vi "Find Center.vi"(7 "Tray Number":dbl format="%#_13g", 9 "XYZTheta":dbl[](array[numeric]), 11 "Gantry In":refnum<k24>) -> (1 "XYZTheta Centers":dbl[][](array[numeric]), 3 "Gantry Out":refnum<k24>)   [LabVIEW 2021, in "Assembly Tray.lvclass"]
uses:
  Assembly Tray.lvclass
  Find Tray.ctl
  Controller/Camera/Machine Vision.ctl
  C:/Program Files (x86)/Aerotech/A3200/LabVIEW/2010/Bin/Aerotech.A3200.dll
  Program Files (x86)/Aerotech/A3200/LabVIEW/2010/Bin/Aerotech.A3200.dll
  Controller/Camera/Image processing.ctl
  Controller/Camera/Camera settings.ctl
  Controller/Camera/Material.ctl
  Program Files (x86)/National Instruments/LabVIEW 2021/examples/Connectivity/Python/support/PythonVersionsEnum.ctl
  Controller/Camera/Camera.lvclass
  Controller/Motion/A3200/A3200.lvclass
  Controller/Motion/Motion.lvclass
panel:
  out "Move by":dbl[](array[numeric])
  in  "Autofiducial (Beta)":bool
  in  "Focus step size":dbl format="%#_13g"
  in  "number of focus steps":i32
  out "Average Strength":dbl
  in  "Focus":bool
  in  "Material":T1
  in  "Camera settings":T2={"Gamma"=1.6, "Gain"=0, "Sharpness"=0, "Contrast"=0.0, "Exposure"=0.0078125} {"Exposure" min=0.000244140625 max=0.5 scale=0.0002..0.5; "Contrast" min=0.0 max=1.0 scale=0.001..1.0; "Sharpness" min=0 max=2 step=1 scale=0.0..2.0; "Gain" min=0 max=100 step=1 scale=0.1..100.0; "Gamma" min=0.01 max=10.0 scale=0.01..10.0}
  in  "Image processing":T3={"Brightness"=128.0, "Contrast"=45.0, "Gamma"=1.0471123} {"Brightness" scale=0.0..400.0; "Contrast" scale=0.0..90.0; "Gamma" scale=0.005..5.0}
  in  "Override presets":bool
  out "Both fiducials recorded":bool
  in  "Machine Vision":T4
  out "Right Fiducial":dbl[](array[numeric]) format="%.6g"
  out "Left Fiducial":dbl[](array[numeric]) format="%.6g"
  out "Gantry":dbl[](array[numeric]) format="%.6g"
  out "Sum":dbl[](array[numeric]) format="%.6g"
  out "Camera":dbl[](array[numeric]) format="%.6g"
  in  "Carrier Tray":T5
  out "Image":T6(plugin-control)
  out "Center":dbl[](array[numeric]) format="%.6g"
  in  "Position Number":i16
  in  "Go to Center":bool
  in  "Calculate":bool
  in  "Record Bottom":bool
  in  "Record Top":bool
  in  "Go to Bottom Fiducial":bool
  in  "Go to Top Fiducial":bool
  in  "Joystick":bool
  in  "Stop":bool
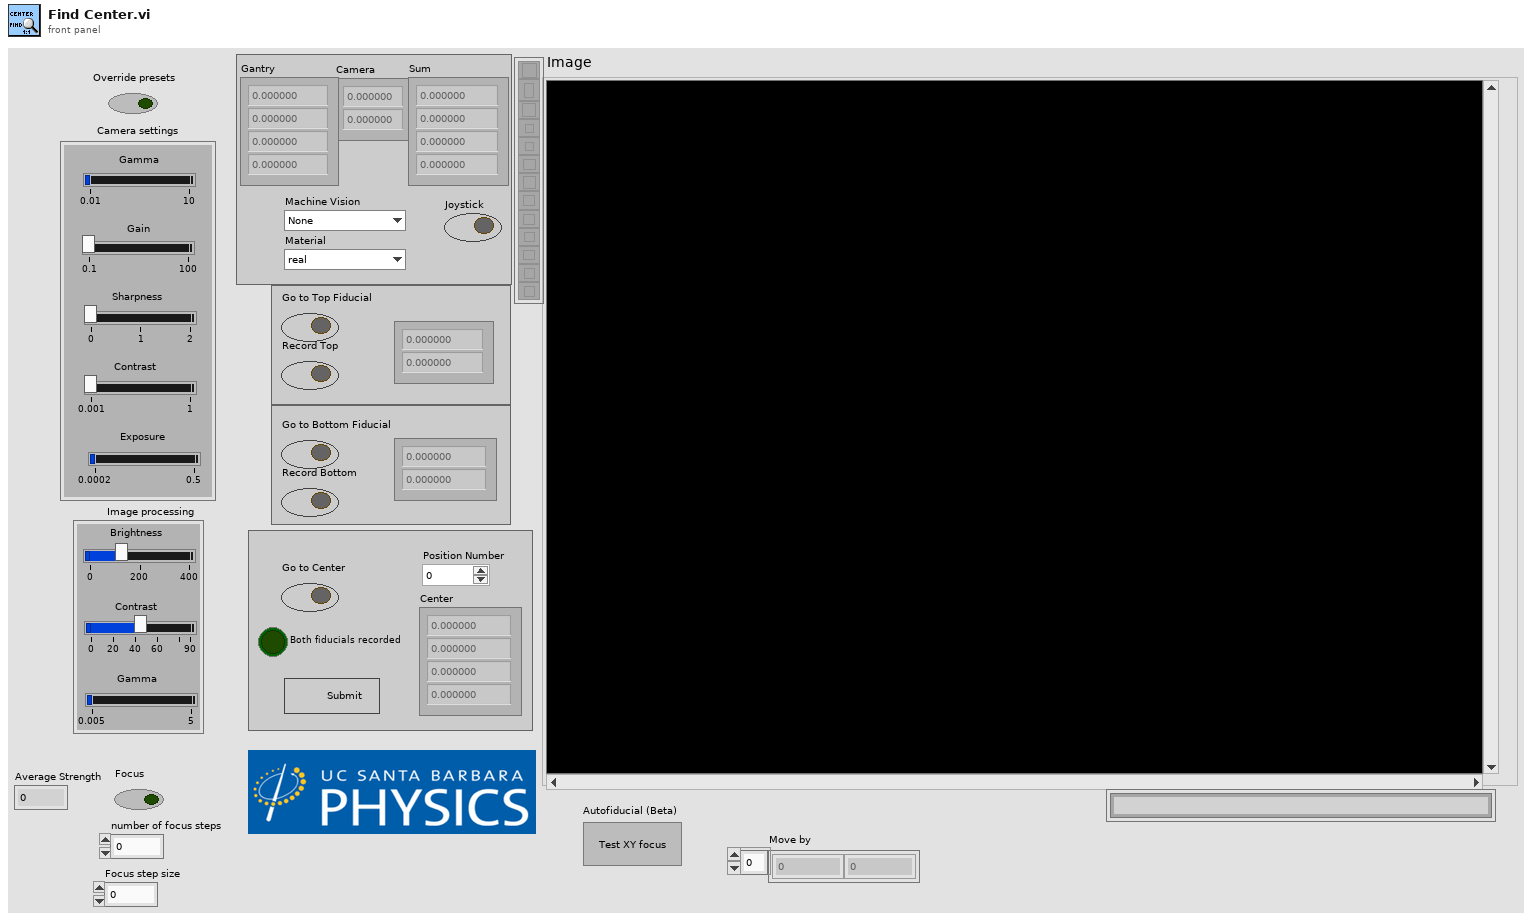
[diagram p1: front panel]
types:
  T1 = typedef "Camera.lvclass/Material.ctl" = enum16{"real", "dummy", "PETG"}
  T2 = typedef "Camera.lvclass/Camera settings.ctl" = cluster{"Gamma":dbl, "Gain":i64, "Sharpness":i64, "Contrast":dbl, "Exposure":dbl}
  T3 = typedef "Camera.lvclass/Image processing.ctl" = cluster{"Brightness":sgl, "Contrast":sgl, "Gamma":sgl}
  T4 = typedef "Camera.lvclass/Machine Vision.ctl" = enum16{"None", "Tray Fiducials", "HPK Silicon", "100um dot", "Hexaboard", "Corner (TL, BR)", "Corner (BL, TR)", "BP gold pad 1", "BP gold pad 2", "BP gold pad 3", "dummy sensor CH2", "dummy sensor CH7", "dummy sensor CH191", "dummy sensor CH197", "sensor box", "sensor circle", "PCB PETG CH2", "PCB PETG CH7", "PCB PETG CH191", "PCB PETG CH197"}
  T5 = typedef "Assembly Tray.lvclass/Find Tray.ctl" = cluster{"Gantry Fiducials":dbl[], "Relative Coordinates":dbl[][], "Camera Fiducials":dbl[][], "XYZTheta Centers":dbl[][], "Workspace Center":dbl[], "Syringe Relative Coordinates":dbl[], "Gantry Region":dbl, "Fiducials":path, "New Fiducials":dbl[][], "Past Fiducials":dbl[][], "XYZTheta":dbl[], "Position":dbl}
  T6 = typedef "IMAQ Image.ctl" = refnum<image>
  T7 = typedef "PythonVersionsEnum.ctl" = enum16{"3.6", "3.7", "3.8", "3.9"}
  T8 = typedef "File Paths.ctl" = cluster{"Glue Pattern Folder":path, "Carrier Tray Folder":path, "Pick Up Tool Fixture Folder":path, "Components Folder":path, "Bellows Tool Offset.txt":path, "Pick Up Tool Offset.txt":path, "Dispense Tip Offset.txt":path, "Log Files":path, "Gantry Assembly Map.txt":path, "Syringe and offset map.txt":path}
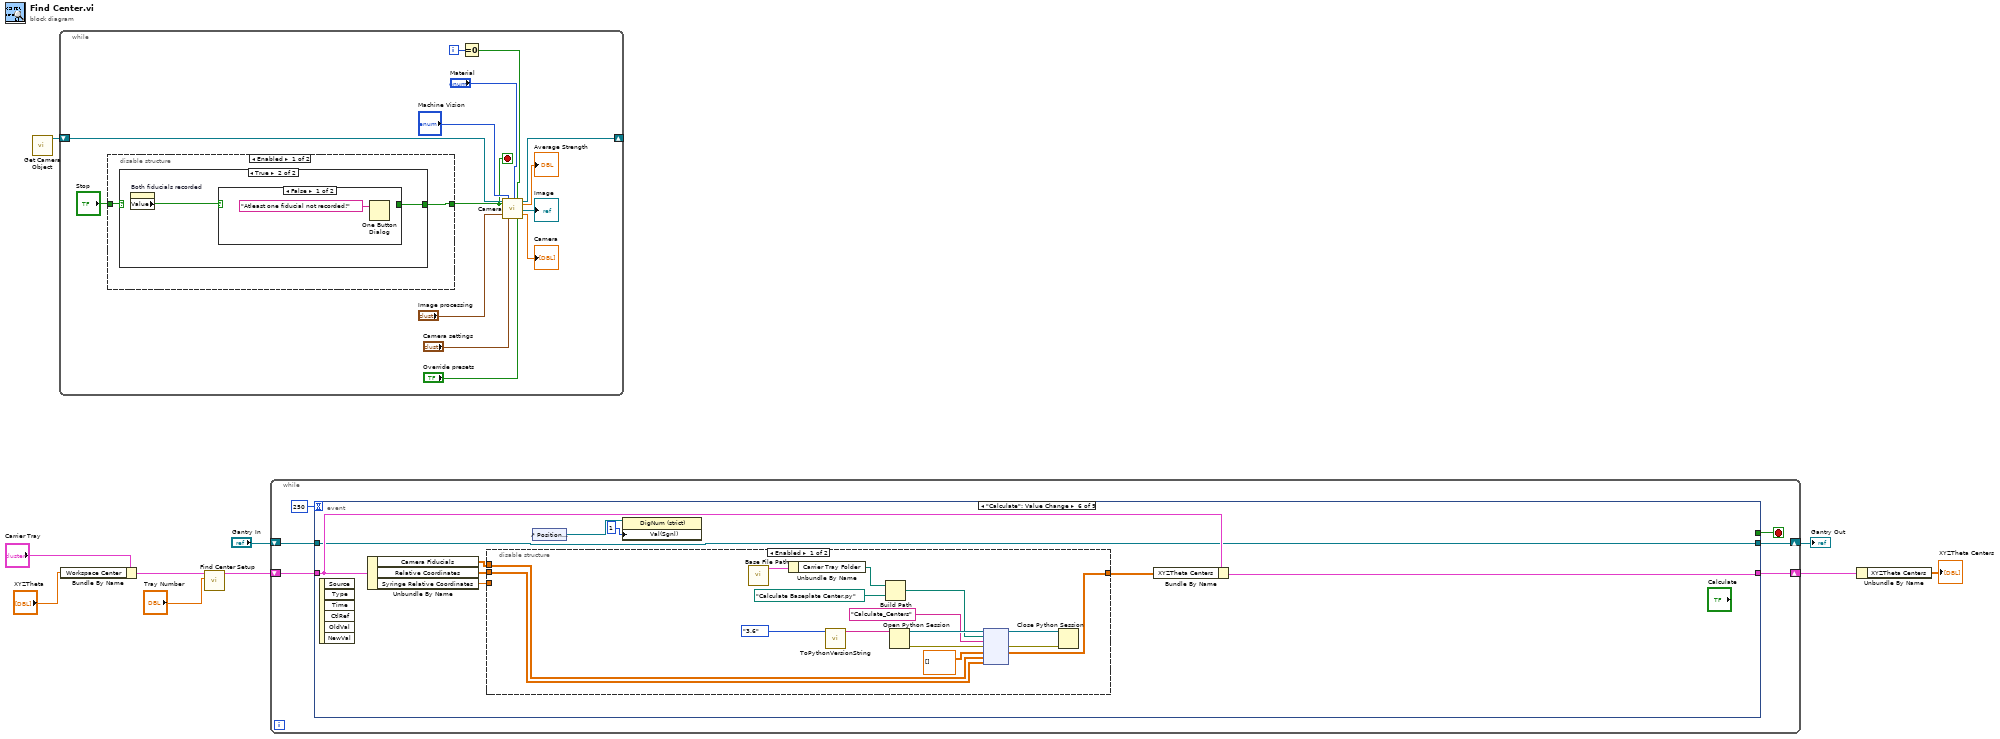
[diagram p0: block diagram]
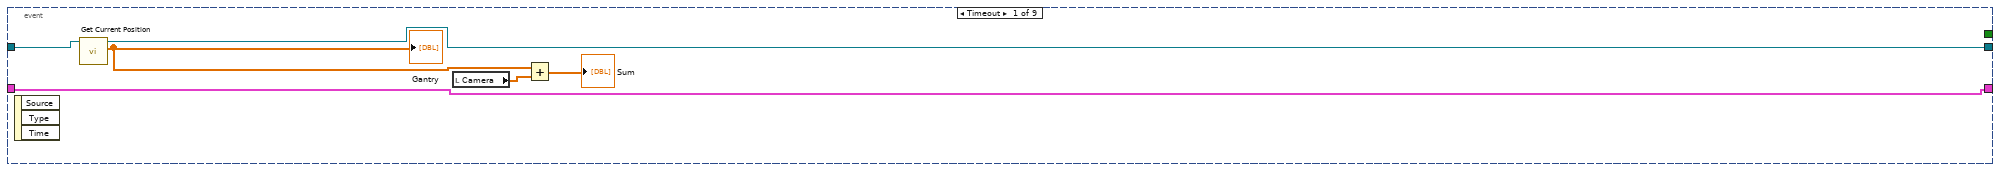
[diagram p2: hidden frame]
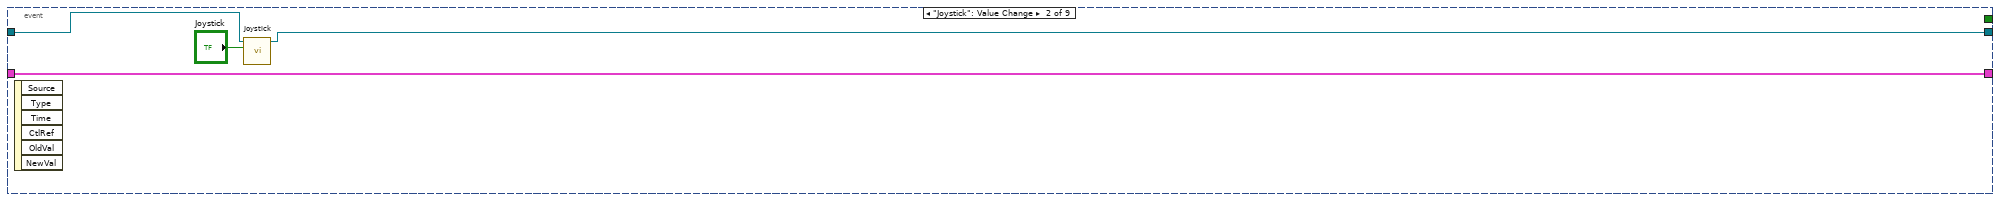
[diagram p3: hidden frame]
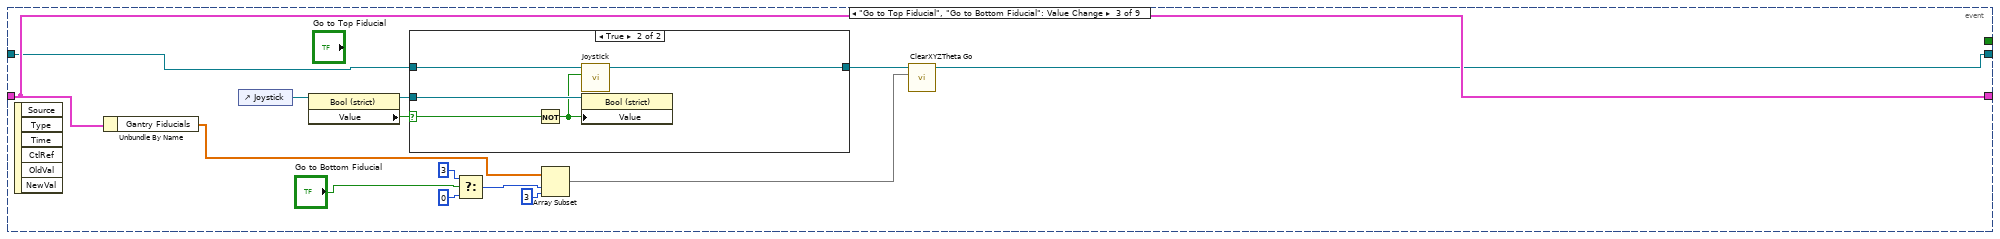
[diagram p4: hidden frame]
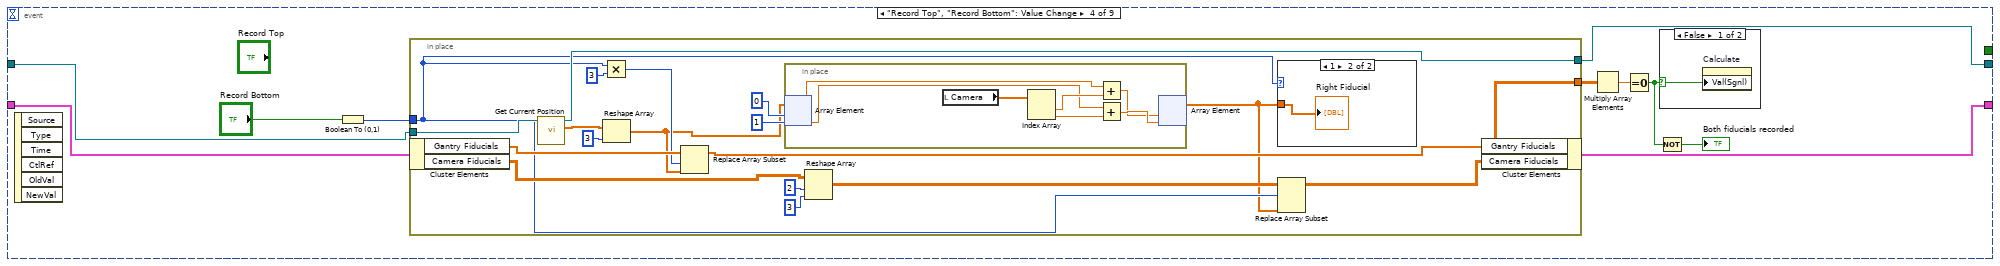
[diagram p6: hidden frame]
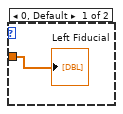
[diagram p8: hidden frame]
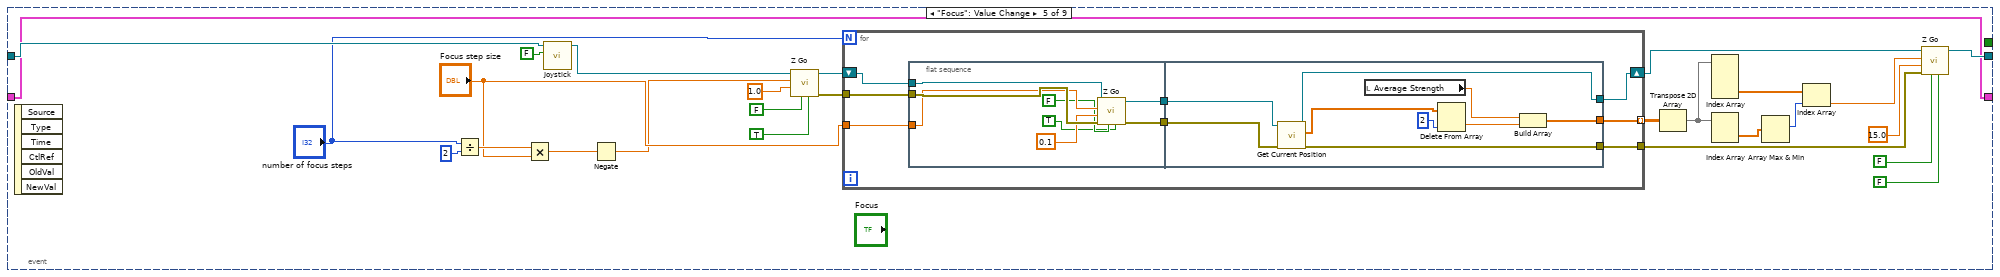
[diagram p9: hidden frame]
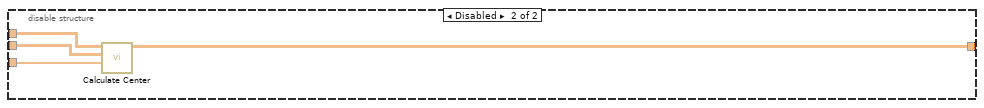
[diagram p10: hidden frame]
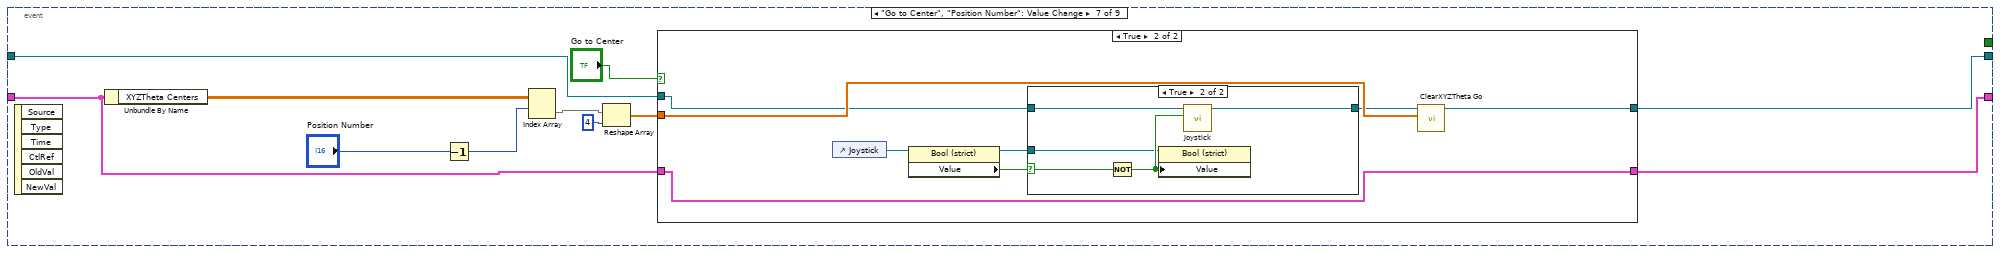
[diagram p11: hidden frame]
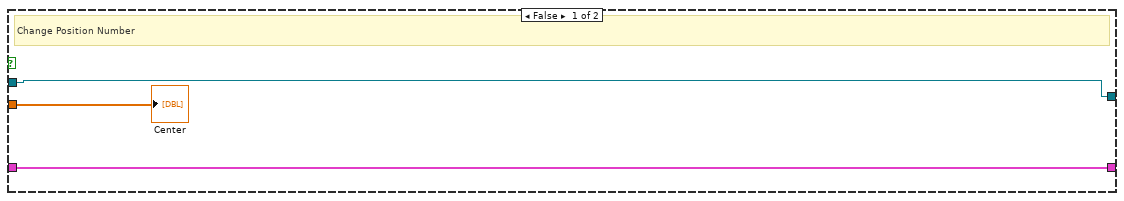
[diagram p12: hidden frame]
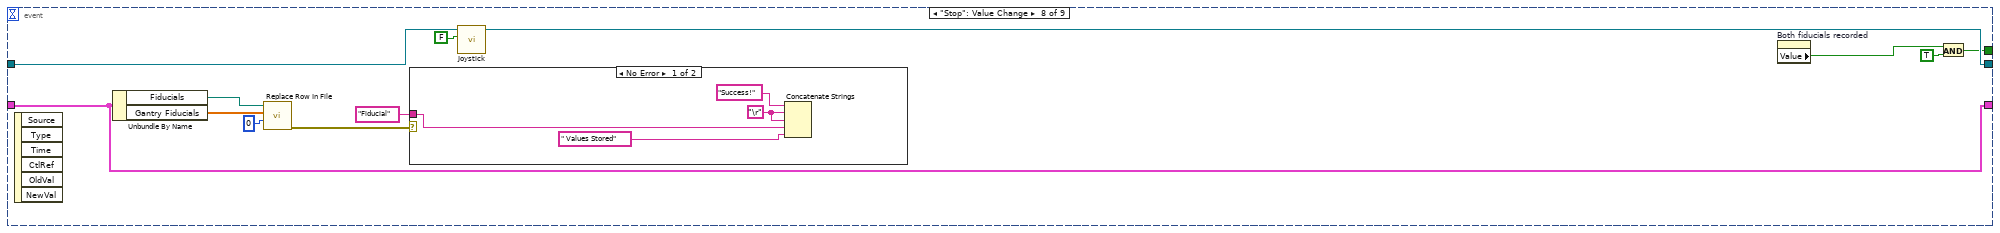
[diagram p14: hidden frame]
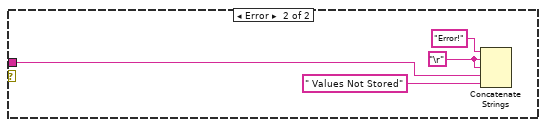
[diagram p15: hidden frame]
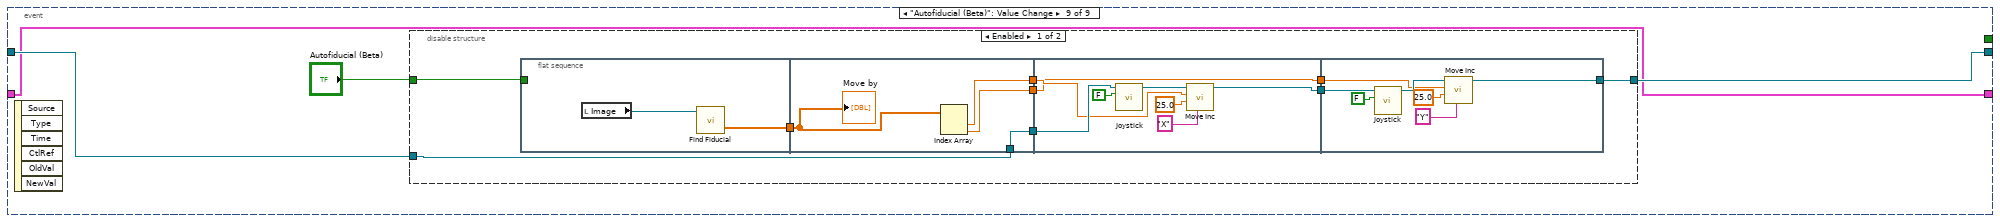
[diagram p16: hidden frame]
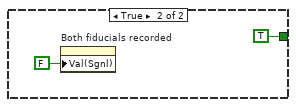
[diagram p19: hidden frame]
diagram:
  n1 = call "Get Camera Object.vi"() -> ("Camera out"=w4:refnum<class "Camera.lvclass">)  [unwired: 10 in, 1 out]
  n2 = while {
    shift-right: [w20] -> _
    shift-left: w4 -> [w24]
    i -> [w14]
    stop <- w19 stop-if-true
    n3 = disable-structure shown="Enabled" {
      disable-tunnel: [w25 w32] -> w19
      disable-tunnel: "Stop" -> [w26 w32]
      frame Enabled {
        n4 = case shown="True" w26 {
          tunnel: [_ w27] -> w25
          frame False {
          }
          frame True {
            n5 = property on="Both fiducials recorded" class="Bool (strict)"() -> ("Value"=w28:bool)  [unwired: 2 in, 2 out]
            n6 = case shown="False" w28 {
              tunnel: [_ TRUE] -> w27
              frame False {
                n7 = One Button Dialog(message="Atleast one fiducial not recorded!") -> ()  [unwired: 1 in, 1 out]
              }
              frame True {
                n8 = property on="Both fiducials recorded" class="Bool (strict)"("Val(Sgnl)"=FALSE) -> ()  [unwired: 2 in, 2 out]
              }
            }
          }
        }
      }
      frame Disabled {
      }
    }
    n9 = Equal To 0?(x=w14) -> (x = 0?=w13:bool)
    n10 = call "Camera.vi"("Camera in"=w24, "Stop"=w19, "BCG Image Processing"="Image processing", "Machine Vision"="Machine Vision", "Camera settings"="Camera settings", "Material"="Material", "Loop 0"=w13, "Override presets"="Override presets") -> ("Camera out"=w20:refnum<class "Camera.lvclass">, "Average Strength"=→"Average Strength":dbl, "Image"=→"Image":T6, "Camera"=→"Camera":dbl[])  [unwired: 5 in, 3 out]
  }
  n11 = Bundle By Name(cluster="Carrier Tray", "Workspace Center"="XYZTheta") -> (w7:T5)
  n12 = call "Find Center Setup.vi"("Carrier Tray"=w7, "Tray Number"="Tray Number") -> ("Assembly Tray Out"=w10:T5)  [unwired: 8 in]
  n13 = while {
    shift-right: [w37] -> w9
    shift-left: w10 -> [w38]
    shift-right: [w33] -> w2
    shift-left: "Gantry In" -> [w34]
    stop <- w36 stop-if-true
    n14 = event shown="[5] \"Calculate\": Value Change" {
      selector: _ -> [_ _ _ _ _ _ _ _ _]
      dyn-events: _ -> [_ _ _ _ _ _ _ _ _]
      timeout: 250 -> [_ _ _ _ _ _ _ _ _]
      tunnel: [w42 w48 w62 w78 w118 w164 w194 w222 w235] -> w37
      tunnel: w38 -> [w42 w48 w62 w73 w118 w165 w195 w222 w235]
      tunnel: [_ _ _ _ _ _ _ w217 _] -> w36
      tunnel: w34 -> [w41 w47 w54 w72 w120 w163 w192 w223 w237]
      tunnel: [w39 w45 w51 w71 w119 w163 w188 w218 w238] -> w33
      event Timeout {
        n15 = event-data() -> ()  [unwired: 1 in, 3 out]
        n16 = call "Get Current Position.vi"("Gantry In"=w41) -> ("XYZTheta Out"=w40:dbl[], "Gantry Out"=w39:refnum<k24>)  [unwired: 8 in, 1 out]
        "Gantry" <- w40
        n17 = local read "Camera"() -> (w44:dbl[])
        n18 = Add(x=w40, y=w44) -> (x+y=→"Sum":dbl[])
      }
      event "Joystick": Value Change {
        n19 = event-data() -> ()  [unwired: 1 in, 6 out]
        n20 = call "Joystick.vi"("Joystick"="Joystick", "Gantry In"=w47) -> ("Gantry Out"=w45:refnum<k24>)  [unwired: 8 in, 1 out]
      }
      event "Go to Top Fiducial", "Go to Bottom Fiducial": Value Change {
        n21 = event-data() -> ()  [unwired: 1 in, 6 out]
        n22 = Unbundle By Name(w62) -> ("Gantry Fiducials"=w50:dbl[])
        n23 = control-ref of="Joystick"() -> (w61:refnum<vi>)
        n24 = property class="Bool (strict)"(reference=w61) -> (reference out=w52:refnum<vi>, "Value"=w55:bool)  [unwired: 1 in, 1 out]
        n25 = case shown="True" w55 {
          selector: w55 -> [_ w68]
          tunnel: w54 -> [w63 w66]
          tunnel: [w63 w65] -> w53
          tunnel: w52 -> [_ w67]
          frame False {
          }
          frame True {
            n26 = Not(x=w68) -> (.not. x?=w64:bool)
            n27 = call "Joystick.vi"("Joystick"=w64, "Gantry In"=w66) -> ("Gantry Out"=w65:refnum<k24>)  [unwired: 8 in, 1 out]
            n28 = property class="Bool (strict)"(reference=w67, "Value"=w64) -> ()  [unwired: 1 in, 2 out]
          }
        }
        n29 = Select(t=3, s="Go to Bottom Fiducial", f=0) -> (s? t:f=w59:i32)
        n30 = Array Subset(array=w50, index=w59, length=3) -> (w49:dbl[])
        n31 = call "ClearXYZTheta Go.vi"("XYZTheta In"=w49, "Gantry In"=w53) -> ("Gantry Out"=w51:refnum<k24>)  [unwired: 7 in, 2 out]
      }
      event "Record Top", "Record Bottom": Value Change {
        n32 = event-data() -> ()  [unwired: 1 in, 6 out]
        n33 = Boolean To (0,1)(Boolean="Record Bottom") -> (0, 1=w75:i16)
        n34 = in-place {
          in-place-border: [w91] -> w76
          in-place-border: w75 -> [w84]
          in-place-border: w72 -> [w86]
          in-place-border: [w85] -> w71
          n35 = in-place-cluster #1(w73) -> ("Gantry Fiducials"=w88:dbl[], "Camera Fiducials"=w95:dbl[][])
          n36 = call "Get Current Position.vi"("Gantry In"=w86) -> ("XYZTheta Out"=w89:dbl[], "Gantry Out"=w85:refnum<k24>)  [unwired: 8 in, 1 out]
          n37 = Multiply(x=w84, y=i16 3) -> (x*y=w82:i16)
          n38 = Reshape Array(w89, 3 ("dimension size")) -> (w81:dbl[])
          n39 = Replace Array Subset(array=w88, new element=w81, index=w82) -> (w87:dbl[])
          n40 = in-place {
            n41 = in-place-array #2(w81, 0, 1) -> (w103:dbl, w101:dbl)
            n42 = local read "Camera"() -> (w104:dbl[])
            n43 = Index Array(array=w104) -> (element #1=w102:dbl, element #2=w100:dbl)  [unwired: 2 in]
            n44 = Add(x=w103, y=w102) -> (x+y=w98:dbl)
            n45 = Add(x=w101, y=w100) -> (x+y=w99:dbl)
            n46 = in-place-array #2(w98, w99) -> (w80:dbl[])  [unwired: 2 out]
          }
          n47 = Reshape Array(w95, 2 ("length"), 3 ("dimension size")) -> (w94:dbl[][])
          n48 = case shown="1" w84 {
            tunnel: w80 -> [w105 w106]
            frame 0, Default {
              "Left Fiducial" <- w105
            }
            frame 1 {
              "Right Fiducial" <- w106
            }
          }
          n49 = Replace Array Subset(array=w94, new element=w80, index (row)=w84) -> (w91:dbl[][])  [unwired: 1 in]
          n50 = in-place-cluster #1("Gantry Fiducials"=w87, "Camera Fiducials"=w91) -> (w78:T5)
        }
        n51 = Multiply Array Elements(1:w76) -> (0:w77:dbl)
        n52 = Equal To 0?(x=w77) -> (x = 0?=w70:bool)
        n53 = Not(x=w70) -> (.not. x?=→"Both fiducials recorded":bool)
        n54 = case shown="False" w70 {
          selector: w70 -> [w79 _]
          frame False {
            n55 = property on="Calculate" class="Bool (strict)"("Val(Sgnl)"=w79) -> ()  [unwired: 2 in, 2 out]
          }
          frame True {
          }
        }
      }
      event "Focus": Value Change {
        n56 = event-data() -> ()  [unwired: 1 in, 6 out]
        n57 = Divide(x="number of focus steps", y=2) -> (x/y=w122:dbl)
        n58 = Multiply(x=w122, y="Focus step size") -> (x*y=w121:dbl)
        n59 = call "Joystick.vi"("Joystick"=FALSE, "Gantry In"=w120) -> ("Gantry Out"=w114:refnum<k24>)  [unwired: 8 in, 1 out]
        n60 = Negate(x=w121) -> (-x=w112:dbl)
        n61 = call "Z Go.vi"("Increment"=TRUE, "Return Immediately"=FALSE ("Increment"), "Speed In"=1.0 ("Speed"), "Position In"=w112, "Gantry In"=w114) -> ("error out"=w109:errorcluster, "Gantry Out"=w113:refnum<k24>)  [unwired: 3 in, 2 out]
        n62 = for {
          N: "number of focus steps" -> [_]
          tunnel: [w138] -> w132 mode=indexing
          tunnel: w109 -> [w137]
          tunnel: [w135] -> w125
          shift-right: [w139] -> w126
          shift-left: w113 -> [w141]
          tunnel: "Focus step size" -> [w134]
          n63 = flat-sequence {
            tunnel: w141 -> [w149]
            tunnel: [w148] -> w140
            tunnel: w137 -> [w146]
            tunnel: [w147] -> w136
            tunnel: w134 -> [w144]
            tunnel: w140 -> [w158]
            tunnel: [w157] -> w139
            tunnel: [w156] -> w138
            tunnel: w136 -> [w152]
            tunnel: [w151] -> w135
            frame #0 {
              n64 = call "Z Go.vi"("Increment"=TRUE, "Return Immediately"=FALSE ("Increment"), "error in (no error)"=w146, "Speed In"=0.1 ("Speed"), "Position In"=w144, "Gantry In"=w149) -> ("error out"=w147:errorcluster, "Gantry Out"=w148:refnum<k24>)  [unwired: 2 in, 2 out]
            }
            frame #1 {
              n65 = call "Get Current Position.vi"("error in (no error)"=w152, "Gantry In"=w158) -> ("error out"=w151:errorcluster, "XYZTheta Out"=w155:dbl[], "Gantry Out"=w157:refnum<k24>)  [unwired: 7 in]
              n66 = local read "Average Strength"() -> (w150:dbl)
              n67 = Delete From Array(array=w155, index=2) -> (deleted portion=w153:dbl)  [unwired: 1 in, 1 out]
              n68 = Build Array(w150, w153) -> (w156:dbl[])
            }
          }
        }
        n69 = Transpose 2D Array(2D array=w132) -> (transposed array=w131:dbl[][])
        n70 = Index Array(array=w131) -> (element #2=w130:dbl[])  [unwired: 4 in, 1 out]
        n71 = Index Array(array=w131) -> (element=w133:dbl[])  [unwired: 2 in]
        n72 = Array Max & Min(array=w133) -> (max index (indices)=w129:i32)  [unwired: 3 out]
        n73 = Index Array(array=w130, index=w129) -> (element=w128:dbl)
        n74 = call "Z Go.vi"("Increment"=FALSE, "Return Immediately"=FALSE ("Increment"), "error in (no error)"=w125, "Speed In"=15.0 ("Speed"), "Position In"=w128, "Gantry In"=w126) -> ("Gantry Out"=w119:refnum<k24>)  [unwired: 2 in, 3 out]
      }
      event "Calculate": Value Change {
        n75 = event-data() -> ()  [unwired: 1 in, 6 out]
        n76 = Unbundle By Name(w165) -> ("Camera Fiducials"=w160:dbl[][], "Relative Coordinates"=w161:dbl[][], "Syringe Relative Coordinates"=w162:dbl[])
        n77 = disable-structure shown="Enabled" {
          disable-tunnel: w160 -> [w171 w185]
          disable-tunnel: w161 -> [w168 w184]
          disable-tunnel: w162 -> [_ w183]
          disable-tunnel: [w172 w186] -> w159
          frame Enabled {
            n78 = call "Base File Path.vi"() -> ("Paths Out"=w170:T8)  [unwired: 11 in]
            n79 = Unbundle By Name(w170) -> ("Carrier Tray Folder"=w169:path)
            n80 = call "ToPythonVersionString.vi"("python version"=PythonVersionsEnum."3.6") -> ("python version string"=w181:string)  [unwired: 10 in]
            n81 = Build Path(base path=w169, name or relative path=path "Calculate Baseplate Center.py") -> (appended path=w174:path)
            n82 = Open Python Session(python version=w181) -> (session out=w180:refnum<k35>, error out=w178:errorcluster)  [unwired: 2 in]
            n83 = node(w180, w174, "Calculate_Centers" ("function name"), w178, dbl[][] [], w171, w168) -> (w179:refnum<k35>, w177:errorcluster, w172:dbl[][])  [unwired: 2 in, 2 out]
            n84 = Close Python Session(session in=w179, error in=w177) -> ()  [unwired: 1 out]
          }
          frame Disabled {
            n85 = call "Calculate Center.vi"("Syringe Coordinates"=w183, "Relative Coordinates"=w184, "Fiducial Measurements"=w185) -> ("XYZTheta Centers"=w186:dbl[][])  [unwired: 8 in]
          }
        }
        n86 = control-ref of="Position Number"() -> (w167:refnum<vi>)
        n87 = property class="DigNum (strict)"(reference=w167, "Val(Sgnl)"=i16 1 ("Value (Signaling)")) -> ()  [unwired: 1 in, 2 out]
        n88 = Bundle By Name(cluster=w165, "XYZTheta Centers"=w159) -> (w164:T5)
      }
      event "Go to Center", "Position Number": Value Change {
        n89 = event-data() -> ()  [unwired: 1 in, 6 out]
        n90 = Unbundle By Name(w195) -> ("XYZTheta Centers"=w187:dbl[][])
        n91 = Decrement(x="Position Number") -> (x-1=w196:i16)
        n92 = Index Array(array=w187, index (row)=w196) -> (element=w190:dbl[])  [unwired: 1 in]
        n93 = Reshape Array(w190, u32 4) -> (w189:dbl[])
        n94 = case shown="True" "Go to Center" {
          tunnel: w189 -> [w200 w206]
          tunnel: w195 -> [w199 w208]
          tunnel: [w199 w208] -> w194
          tunnel: w192 -> [w198 w202]
          tunnel: [w198 w207] -> w188
          frame False {
            # "Change Position Number"
            "Center" <- w200
          }
          frame True {
            n95 = control-ref of="Joystick"() -> (w205:refnum<vi>)
            n96 = property class="Bool (strict)"(reference=w205) -> (reference out=w203:refnum<vi>, "Value"=w204:bool)  [unwired: 1 in, 1 out]
            n97 = case shown="True" w204 {
              selector: w204 -> [_ w214]
              tunnel: w202 -> [w209 w213]
              tunnel: [w209 w212] -> w201
              tunnel: w203 -> [_ w210]
              frame False {
              }
              frame True {
                n98 = Not(x=w214) -> (.not. x?=w211:bool)
                n99 = property class="Bool (strict)"(reference=w210, "Value"=w211) -> ()  [unwired: 1 in, 2 out]
                n100 = call "Joystick.vi"("Joystick"=w211, "Gantry In"=w213) -> ("Gantry Out"=w212:refnum<k24>)  [unwired: 8 in, 1 out]
              }
            }
            n101 = call "ClearXYZTheta Go.vi"("XYZTheta In"=w206, "Gantry In"=w201) -> ("Gantry Out"=w207:refnum<k24>)  [unwired: 7 in, 2 out]
          }
        }
      }
      event "Stop": Value Change {
        n102 = event-data() -> ()  [unwired: 1 in, 6 out]
        n103 = Unbundle By Name(w222) -> ("Fiducials"=w220:path, "Gantry Fiducials"=w221:dbl[])
        n104 = call "Replace Row In File.vi"("Index"=0, "Insert Array"=w221, "Path"=w220) -> ("error out"=w226:errorcluster)  [unwired: 8 in]
        n105 = case shown="No Error" w226 {
          tunnel: "Fiducial" -> [w227 w234]
          frame No Error {
            w228 = "\r"
            n106 = Concatenate Strings("Success!", w228, w228, w227, " Values Stored") -> ()  [unwired: 1 out]
          }
          frame Error {
            w231 = "\r"
            n107 = Concatenate Strings("Error!", w231, w231, w234, " Values Not Stored") -> ()  [unwired: 1 out]
          }
        }
        n108 = call "Joystick.vi"("Joystick"=FALSE, "Gantry In"=w223) -> ("Gantry Out"=w218:refnum<k24>)  [unwired: 8 in, 1 out]
        n109 = property on="Both fiducials recorded" class="Bool (strict)"() -> ("Value"=w215:bool)  [unwired: 2 in, 2 out]
        n110 = And(x=w215, y=TRUE) -> (x .and. y?=w217:bool)
      }
      event "Autofiducial (Beta)": Value Change {
        n111 = event-data() -> ()  [unwired: 1 in, 6 out]
        n112 = disable-structure shown="Enabled" {
          disable-tunnel: [w242 w269] -> w238
          disable-tunnel: w237 -> [w241 w269]
          disable-tunnel: "Autofiducial (Beta)" -> [w240 _]
          frame Enabled {
            n113 = flat-sequence {
              tunnel: w240 -> [_]
              tunnel: [w248] -> w239
              tunnel: w241 -> [w253]
              tunnel: [w253] -> w247
              tunnel: [w252] -> w246
              tunnel: [w251] -> w245
              tunnel: w239 -> [w250]
              tunnel: w247 -> [w257]
              tunnel: [w256] -> w244
              tunnel: w246 -> [w255]
              tunnel: [w254] -> w243
              tunnel: w245 -> [w254]
              tunnel: [w263] -> w242
              tunnel: w244 -> [w264]
              tunnel: w243 -> [w262]
              frame #0 {
                n114 = local read "Image"() -> (w249:T6)
                n115 = call "Find Fiducial.vi"("Image"=w249) -> ("Move by (mm)"=w248:dbl[])  [unwired: 3 in]
              }
              frame #1 {
                n116 = Index Array(array=w250) -> (element #1=w252:dbl, element #2=w251:dbl)  [unwired: 2 in]
                "Move by" <- w250
              }
              frame #2 {
                n117 = call "Joystick.vi"("Joystick"=FALSE, "Gantry In"=w257) -> ("Gantry Out"=w258:refnum<k24>)  [unwired: 8 in, 1 out]
                n118 = call "Move Inc.vi"("Axis"="X", "Speed"=25.0, "Distance"=w255, "Gantry In"=w258) -> ("Gantry Out"=w256:refnum<k24>)  [unwired: 6 in, 1 out]
              }
              frame #3 {
                n119 = call "Joystick.vi"("Joystick"=FALSE, "Gantry In"=w264) -> ("Gantry Out"=w265:refnum<k24>)  [unwired: 8 in, 1 out]
                n120 = call "Move Inc.vi"("Axis"="Y", "Speed"=25.0, "Distance"=w262, "Gantry In"=w265) -> ("Gantry Out"=w263:refnum<k24>)  [unwired: 6 in, 1 out]
              }
            }
          }
          frame Disabled {
          }
        }
      }
    }
  }
  "Gantry Out" <- w2
  n121 = Unbundle By Name(w9) -> ("XYZTheta Centers"=→"XYZTheta Centers":dbl[][])
